vi "Show Data Logger.vi"(8 "error in":errorcluster, 11 "Series Actor in":refnum<class "Series Actor.lvclass">) -> (0 "error out":errorcluster, 3 "Series Actor out":refnum<class "Series Actor.lvclass">)   [LabVIEW 2023, in "Series Actor.lvlib" / "Series Actor.lvclass"]
uses:
  Series Actor.lvclass
  Series Actor.lvclass/Series Actor.ctl
  <vilib>/MGI/Panel Manager/Panel Actor/Panel Actor Messages/Show Panel Msg/Show Panel Msg.lvclass
  <vilib>/ActorFramework/Message Enqueuer/Message Enqueuer.lvclass
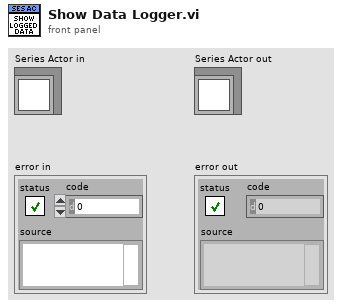
[diagram p1: front panel]
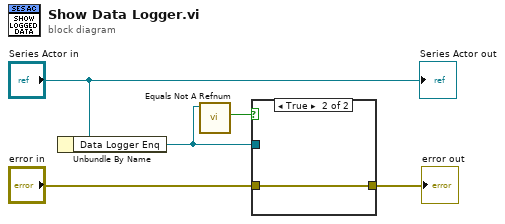
[diagram p0: block diagram]
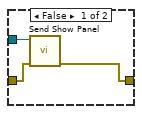
[diagram p2: hidden frame]
diagram:
  n1 = Unbundle By Name("Series Actor in") -> ("Data Logger Enq"=w2:refnum<class "Message Enqueuer.lvclass">)
  n2 = call <vilib>:"Equals Not A Refnum.vi"("Message Enqueuer"=w2) -> ("Not a refnum?"=w3:bool)  [unwired: 10 in]
  n3 = case shown="True" w3 {
    tunnel: w2 -> [w8 _]
    tunnel: "error in" -> [w7 w9]
    tunnel: [w6 w9] -> w4
    frame False {
      n4 = call <vilib>:"Send Show Panel.vi"("Error In"=w7, "Message Enqueuer in"=w8) -> ("Error Out"=w6:errorcluster)  [unwired: 8 in, 1 out]
    }
    frame True {
    }
  }
  "error out" <- w4
  "Series Actor out" <- "Series Actor in"
